vi "数据查询_仪器数据.vi"() -> ()   [LabVIEW 2016]
uses:
  <vilib>/Utility/miscctls.llb/LVRowAndColumnUnsignedTypeDef.ctl
  <vilib>/Utility/miscctls.llb/LVPointTypeDef.ctl
panel:
  in  "工作模式":string(combo)="全部数据"
  in  "查询":bool
  in  "结束日期":string="2020/01/01"
  in  "起始日期":string="2010/01/01"
  in  "组合框":string(combo)
  out "数据表":string[][](table)
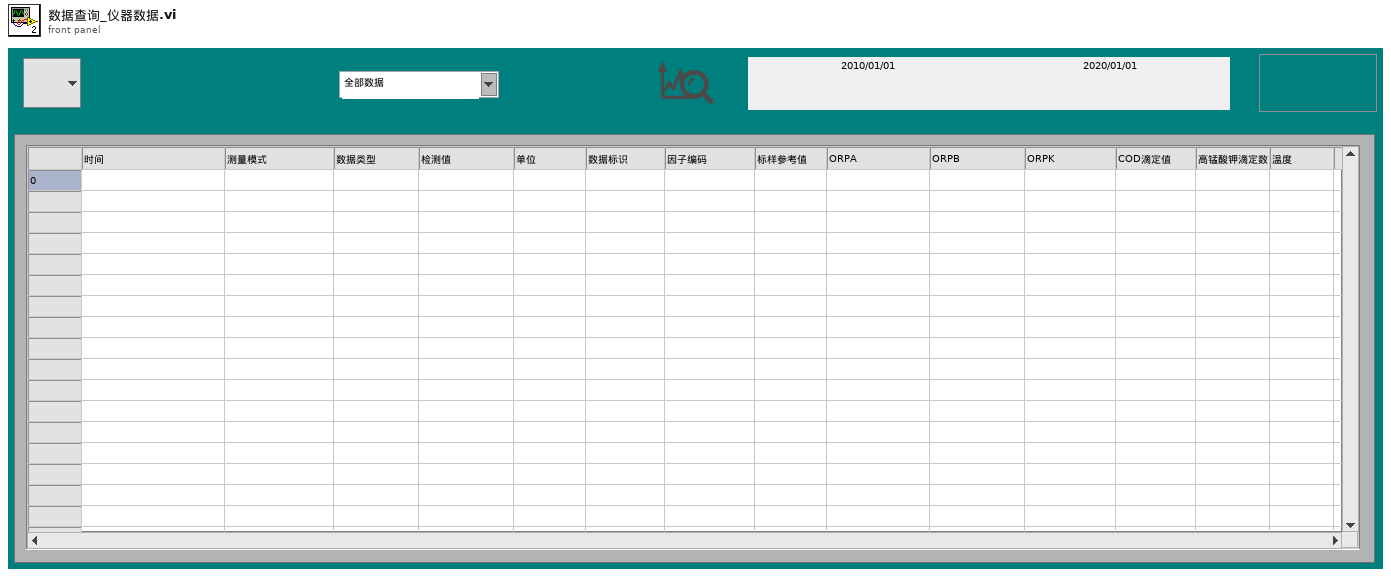
[diagram p1: front panel]
types:
  T1 = enum16{"None", "On Hover", "On Key Focus", "On Hover or Key Focus"}
  T2 = typedef "LVRowAndColumnUnsignedTypeDef.ctl" = cluster{"Row":u32, "Column":u32}
  T3 = typedef "LVPoint32TypeDef.ctl" = cluster{"Horizontal":i32, "Vertical":i32}
  T4 = typedef "LVRowAndColumnTypeDef.ctl" = cluster{"Row":i32, "Column":i32}
  T5 = typedef "LVPointTypeDef.ctl" = cluster{"Horizontal":i16, "Vertical":i16}
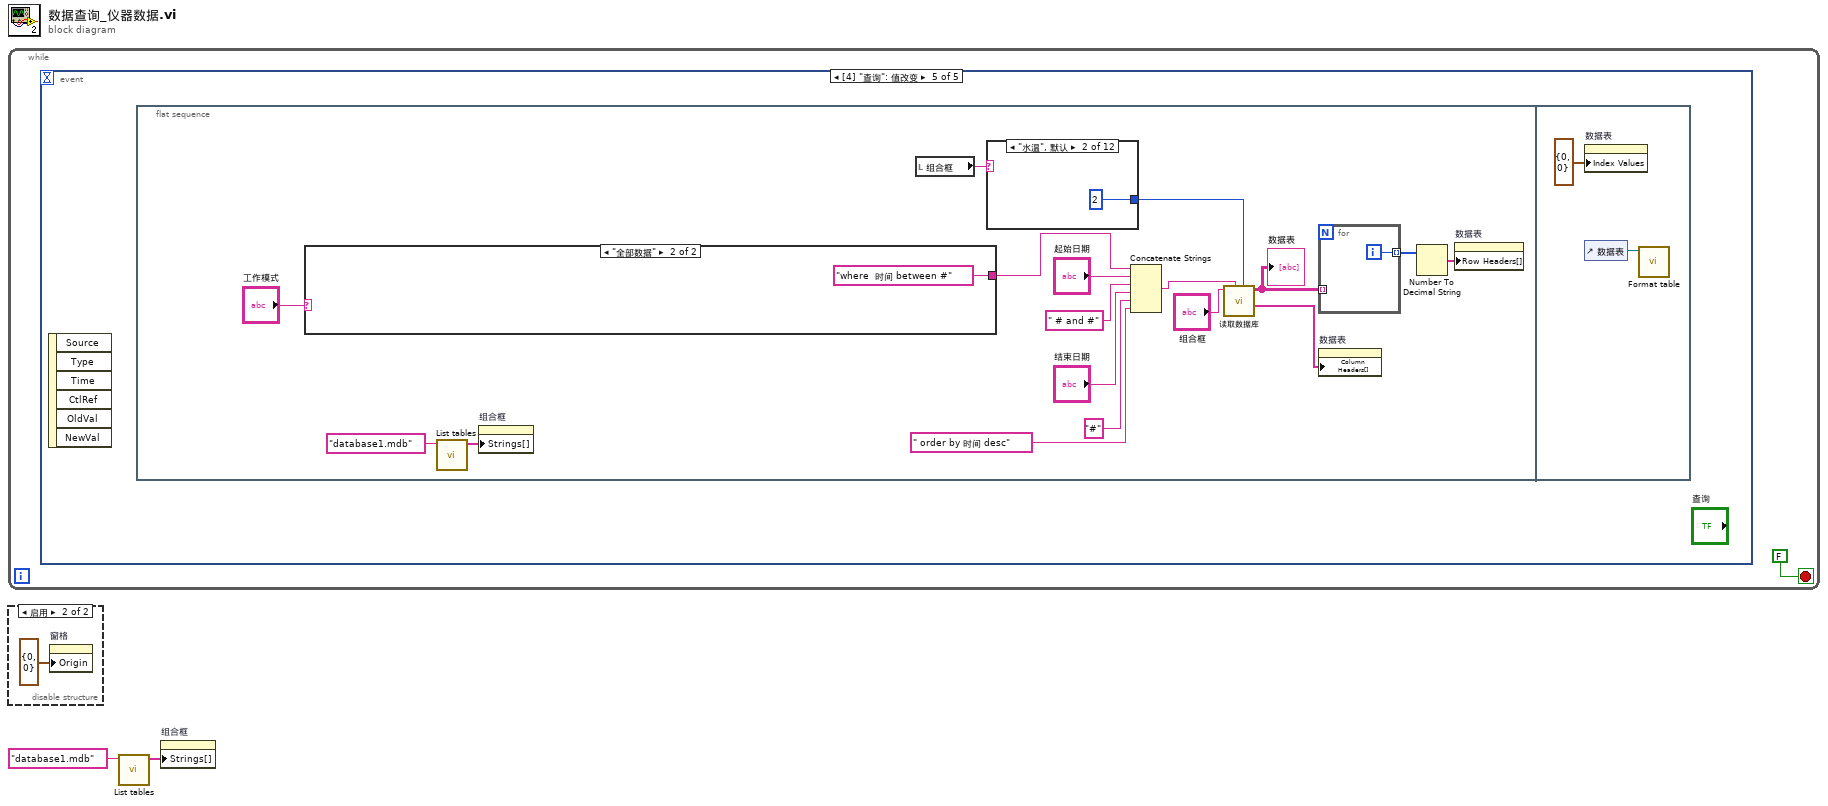
[diagram p0: block diagram]
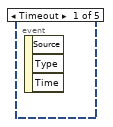
[diagram p2: hidden frame]
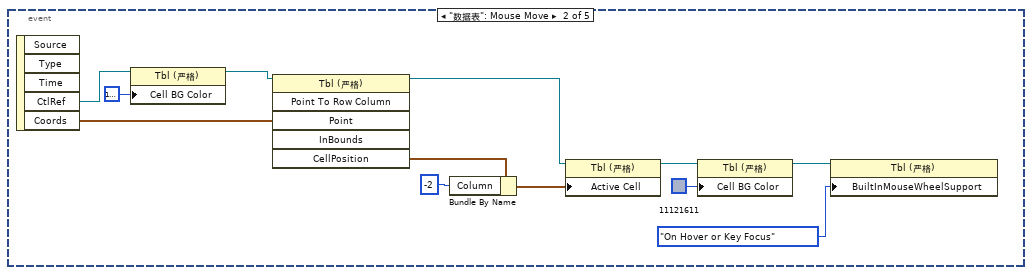
[diagram p3: hidden frame]
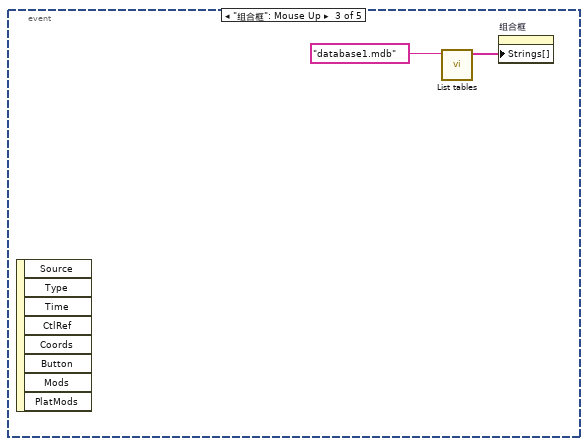
[diagram p4: hidden frame]
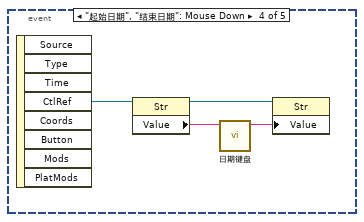
[diagram p5: hidden frame]
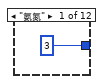
[diagram p6: hidden frame]
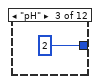
[diagram p7: hidden frame]
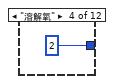
[diagram p8: hidden frame]
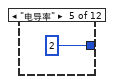
[diagram p9: hidden frame]
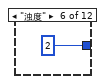
[diagram p10: hidden frame]
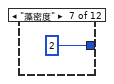
[diagram p11: hidden frame]
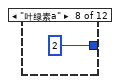
[diagram p12: hidden frame]
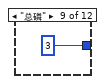
[diagram p13: hidden frame]
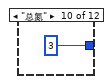
[diagram p14: hidden frame]
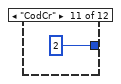
[diagram p15: hidden frame]
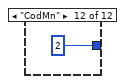
[diagram p16: hidden frame]
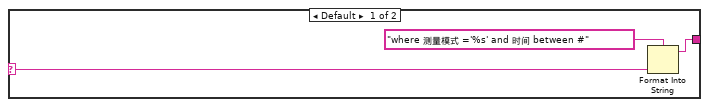
[diagram p17: hidden frame]
diagram:
  n1 = while {
    stop <- FALSE stop-if-true
    n2 = event shown="[4] \"查询\": 值改变" {
      selector: _ -> [_ _ _ _ _]
      dyn-events: _ -> [_ _ _ _ _]
      timeout: _ -> [_ _ _ _ _]
      event Timeout {
        n3 = event-data() -> ()  [unwired: 1 in, 3 out]
      }
      event "数据表": Mouse Move {
        n4 = event-data() -> ("CtlRef"=w6:refnum<vi>, "Coords"=w7:T3)  [unwired: 1 in, 3 out]
        n5 = property class="Tbl (严格)"(reference=w6, "Cell BG Color"=u32 16777225) -> (reference out=w11:refnum<vi>)  [unwired: 1 in, 1 out]
        n6 = invoke class="Tbl (严格)" method="Point To Row Column"(reference=w11, "Point"=w7) -> (reference out=w9:refnum<vi>, "CellPosition"=w8:T4)  [unwired: 4 in, 4 out]
        n7 = Bundle By Name(cluster=w8, "Column"=-2) -> (w15:T4)
        n8 = property class="Tbl (严格)"(reference=w9, "Active Cell"=w15) -> (reference out=w13:refnum<vi>)  [unwired: 1 in, 1 out]
        n9 = property class="Tbl (严格)"(reference=w13, "Cell BG Color"=u32 11121611) -> (reference out=w5:refnum<vi>)  [unwired: 1 in, 1 out]
        n10 = property class="Tbl (严格)"(reference=w5, "BuiltInMouseWheelSupport"=T1."On Hover or Key Focus" ("内置鼠标滑轮支持")) -> ()  [unwired: 1 in, 2 out]
      }
      event "组合框": Mouse Up {
        n11 = event-data() -> ()  [unwired: 1 in, 8 out]
        n12 = call "List tables.vi"("database"="database1.mdb") -> ("tables"=w17:string[])  [unwired: 9 in, 1 out]
        n13 = property on="组合框" class="CmbBox"("Strings[]"=w17) -> ()  [unwired: 2 in, 2 out]
      }
      event "起始日期", "结束日期": Mouse Down {
        n14 = event-data() -> ("CtlRef"=w21:refnum<vi>)  [unwired: 1 in, 7 out]
        n15 = property class="Str"(reference=w21) -> (reference out=w19:refnum<vi>, "Value"=w20:string)  [unwired: 1 in, 1 out]
        n16 = call "日期键盘.vi"("原值"=w20) -> ("x+y"=w18:string)  [unwired: 10 in]
        n17 = property class="Str"(reference=w19, "Value"=w18) -> ()  [unwired: 1 in, 2 out]
      }
      event "查询": Value Change {
        n18 = event-data() -> ()  [unwired: 1 in, 6 out]
        n19 = flat-sequence {
          frame #0 {
            n20 = case shown="\"全部数据\"" "工作模式" {
              selector: "工作模式" -> [w53 _]
              tunnel: [w51 "where  时间 between #" ("condition")] -> w26
              frame Default {
                n21 = Format Into String(format string="where 测量模式 ='%s' and 时间 between #" ("condition"), w53) -> (resulting string=w51:string)  [unwired: 2 in, 1 out]
              }
              frame "全部数据" {
              }
            }
            n22 = call "List tables.vi"("database"="database1.mdb") -> ("tables"=w23:string[])  [unwired: 9 in, 1 out]
            n23 = property on="组合框" class="CmbBox"("Strings[]"=w23) -> ()  [unwired: 2 in, 2 out]
            n24 = local read "组合框"() -> (w25:string)
            n25 = case shown="\"水温\", 默认" w25 {
              tunnel: [i16 3 ("精度(6)") i16 2 ("精度(6)") i16 2 ("精度(6)") i16 2 ("精度(6)") i16 2 ("精度(6)") i16 2 ("精度(6)") i16 2 ("精度(6)") i16 2 ("精度(6)") i16 3 ("精度(6)") i16 3 ("精度(6)") i16 2 ("精度(6)") i16 2 ("精度(6)")] -> w24
              frame "氨氮" {
              }
              frame "水温", Default {
              }
              frame "pH" {
              }
              frame "溶解氧" {
              }
              frame "电导率" {
              }
              frame "浊度" {
              }
              frame "藻密度" {
              }
              frame "叶绿素a" {
              }
              frame "总磷" {
              }
              frame "总氮" {
              }
              frame "CodCr" {
              }
              frame "CodMn" {
              }
            }
            n26 = Concatenate Strings(w26, "起始日期", " # and #" ("condition"), "结束日期", "#" ("condition"), " order by 时间 desc" ("字符串")) -> (w37:string)
            n27 = call "读取数据库.vi"("精度(6)"=w24, "condition"=w37, "组合框"="组合框") -> ("columns"=w33:string[], "表格"=w30:string[][])  [unwired: 5 in, 2 out]
            "数据表" <- w30
            n28 = for {
              tunnel: w30 -> [_] mode=indexing
              tunnel: [w55] -> w29 mode=indexing
              i -> [w55]
            }
            n29 = property on="数据表" class="Tbl (严格)"("Column Headers[]"=w33) -> ()  [unwired: 2 in, 2 out]
            n30 = Number To Decimal String(number=w29) -> (decimal integer string=w28:string[])  [unwired: 1 in]
            n31 = property on="数据表" class="Tbl (严格)"("Row Headers[]"=w28) -> ()  [unwired: 2 in, 2 out]
          }
          frame #1 {
            n32 = property on="数据表" class="Tbl (严格)"("Index Values"=T2 {"Row"=0, "Column"=0} ("索引值")) -> ()  [unwired: 2 in, 2 out]
            n33 = control-ref of="数据表"() -> (w56:refnum<vi>)
            n34 = call "Format table.vi"("Table输入"=w56) -> ()  [unwired: 11 in]
          }
        }
      }
    }
  }
  n35 = disable-structure shown="启用" {
    frame Disabled {
    }
    frame Enabled {
      n36 = property on="窗格" class="Pane"("Origin"=T5 {"Horizontal"=0, "Vertical"=0} ("原点")) -> ()  [unwired: 2 in, 2 out]
    }
  }
  n37 = call "List tables.vi"("database"="database1.mdb") -> ("tables"=w1:string[])  [unwired: 9 in, 1 out]
  n38 = property on="组合框" class="CmbBox"("Strings[]"=w1) -> ()  [unwired: 2 in, 2 out]
